vi "valves_flushrings.vi"(0 "COM4 in":refnum<k24>, 2 "Input solution":dbl=1.0, 3 "Rings to open":u32, 5 "error in":errorcluster) -> (6 "COM4 out":refnum<k24>, 8 "error out":errorcluster)   [LabVIEW 2018]
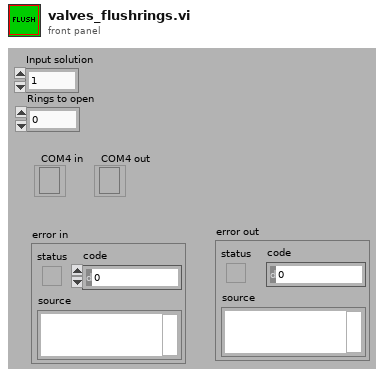
[diagram p1: front panel]
types:
  T1 = cluster{"Op A":u8[], "Op B":u8[], "Op C":u8[], "open":u8[], "L 3 A":u8[], "L 4 A 16":u8[], "F1 A":u8[], "L 4 A 34":u8[], "L 4 A 5":u8[], "FPw1 A":u8[], "L 2 A":u8[], "L 1 C FS":u8[], "L 2 C FS":u8[], "L 4 C 456 FS":u8[], "L 4 C 123 FS":u8[], "L 1 A":u8[], "L 1 C":u8[], "L 2 C":u8[], "L 4 C 456":u8[], "L 4 C 123":u8[], "FPw1 C":u8[], "F1 B":u8[], "F1 C":u8[], "F2 C":u8[], "F5 C":u8[]}
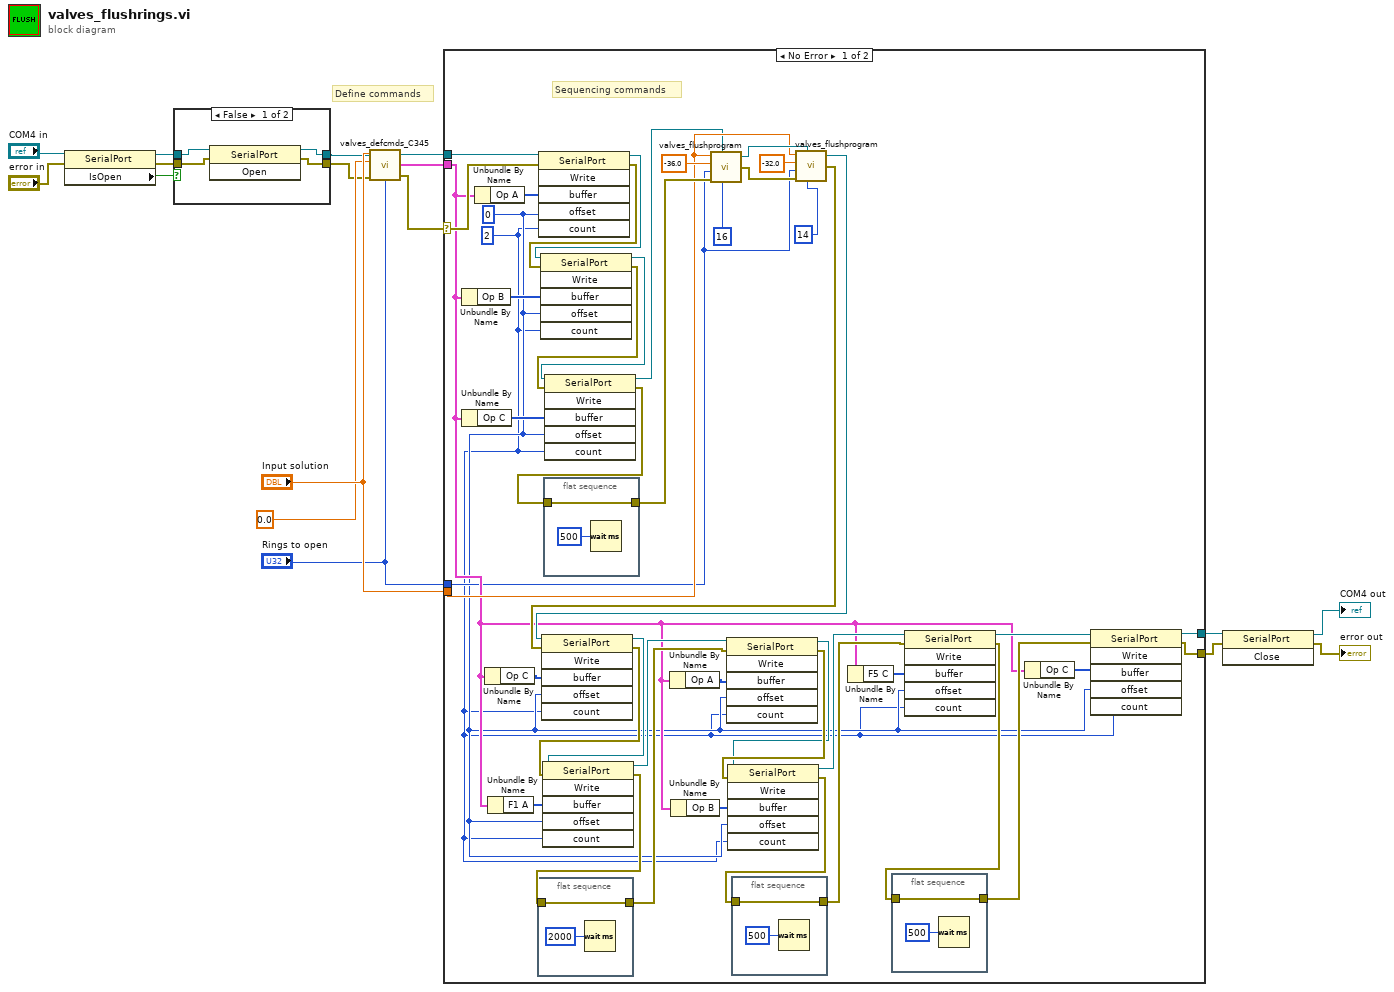
[diagram p0: block diagram]
diagram:
  # "Define commands"
  n1 = property class="SerialPort"(reference="COM4 in", error in="error in") -> (reference out=w9:refnum<k24>, error out=w10:errorcluster, "IsOpen"=w11:bool)
  n2 = case shown="False" w11 {
    tunnel: [w18 w23] -> w7
    tunnel: [w19 w22] -> w6
    tunnel: w10 -> [w20 w22]
    tunnel: w9 -> [w21 w23]
    frame False {
      n3 = invoke class="SerialPort" method="Open"(reference=w21, error in=w20) -> (reference out=w18:refnum<k24>, error out=w19:errorcluster)  [unwired: 1 in, 1 out]
    }
    frame True {
    }
  }
  n4 = call "valves_defcmds_C345.vi"("Input solution"="Input solution", "Add to C"=0.0, "Rings to open"="Rings to open", "error in"=w6, "COM4 in"=w7) -> ("COM4 out"=w15:refnum<k24>, "Commands out"=w16:T1, "error out"=w17:errorcluster)
  n5 = case shown="No Error" w17 {
    selector: w17 -> [w63 w79]
    tunnel: w15 -> [w69 w78]
    tunnel: [w54 w79] -> w4
    tunnel: w16 -> [w38 _]
    tunnel: "Rings to open" -> [w36 _]
    tunnel: "Input solution" -> [w43 _]
    tunnel: [w47 w78] -> w2
    frame No Error {
      w24 = 2 ("count")
      w25 = 0 ("offset")
      # "Sequencing commands"
      n6 = Unbundle By Name(w38) -> ("Op B"=w34:u8[])
      n7 = Unbundle By Name(w38) -> ("Op C"=w33:u8[])
      n8 = Unbundle By Name(w38) -> ("Op A"=w35:u8[])
      n9 = Unbundle By Name(w38) -> ("Op C"=w31:u8[])
      n10 = Unbundle By Name(w38) -> ("F1 A"=w26:u8[])
      n11 = flat-sequence {
        tunnel: [w74] -> w46
        tunnel: w45 -> [w74]
        frame #0 {
          n12 = Wait (ms)(milliseconds to wait=u32 2000) -> ()  [unwired: 1 out]
        }
      }
      n13 = invoke class="SerialPort" method="Write"(reference=w69, error in=w63, "buffer"=w35, "offset"=w25, "count"=w24) -> (reference out=w68:refnum<k24>, error out=w67:errorcluster)  [unwired: 1 in, 4 out]
      n14 = invoke class="SerialPort" method="Write"(reference=w68, error in=w67, "buffer"=w34, "offset"=w25, "count"=w24) -> (reference out=w66:refnum<k24>, error out=w65:errorcluster)  [unwired: 1 in, 4 out]
      n15 = flat-sequence {
        tunnel: [w76] -> w62
        tunnel: w64 -> [w76]
        frame #0 {
          n16 = Wait (ms)(milliseconds to wait=u32 500) -> ()  [unwired: 1 out]
        }
      }
      n17 = invoke class="SerialPort" method="Write"(reference=w66, error in=w65, "buffer"=w33, "offset"=w25, "count"=w24) -> (reference out=w32:refnum<k24>, error out=w64:errorcluster)  [unwired: 1 in, 4 out]
      n18 = Unbundle By Name(w38) -> ("Op A"=w30:u8[])
      n19 = Unbundle By Name(w38) -> ("Op B"=w27:u8[])
      n20 = call "valves_flushprogram.vi"("Input solution"=w43, "COM4 in"=w32, "Add to C"=-36.0, "Rings to open"=w36, "Cycles"=16 ("Input solution"), "error in"=w62) -> ("COM4 out"=w59:refnum<k24>, "error out"=w58:errorcluster)  [unwired: 1 in]
      n21 = flat-sequence {
        tunnel: [w72] -> w41
        tunnel: w42 -> [w72]
        frame #0 {
          n22 = Wait (ms)(milliseconds to wait=u32 500) -> ()  [unwired: 1 out]
        }
      }
      n23 = call "valves_flushprogram.vi"("Input solution"=w43, "COM4 in"=w59, "Add to C"=-32.0, "Rings to open"=w36, "Cycles"=14 ("Input solution"), "error in"=w58) -> ("COM4 out"=w53:refnum<k24>, "error out"=w57:errorcluster)  [unwired: 1 in]
      n24 = invoke class="SerialPort" method="Write"(reference=w53, error in=w57, "buffer"=w31, "offset"=w25, "count"=w24) -> (reference out=w52:refnum<k24>, error out=w56:errorcluster)  [unwired: 1 in, 4 out]
      n25 = invoke class="SerialPort" method="Write"(reference=w52, error in=w56, "buffer"=w26, "offset"=w25, "count"=w24) -> (reference out=w51:refnum<k24>, error out=w45:errorcluster)  [unwired: 1 in, 4 out]
      n26 = invoke class="SerialPort" method="Write"(reference=w51, error in=w46, "buffer"=w30, "offset"=w25, "count"=w24) -> (reference out=w50:refnum<k24>, error out=w55:errorcluster)  [unwired: 1 in, 4 out]
      n27 = invoke class="SerialPort" method="Write"(reference=w50, error in=w55, "buffer"=w27, "offset"=w25, "count"=w24) -> (reference out=w49:refnum<k24>, error out=w42:errorcluster)  [unwired: 1 in, 4 out]
      n28 = Unbundle By Name(w38) -> ("F5 C"=w29:u8[])
      n29 = flat-sequence {
        tunnel: [w70] -> w39
        tunnel: w40 -> [w70]
        frame #0 {
          n30 = Wait (ms)(milliseconds to wait=u32 500) -> ()  [unwired: 1 out]
        }
      }
      n31 = invoke class="SerialPort" method="Write"(reference=w49, error in=w41, "buffer"=w29, "offset"=w25, "count"=w24) -> (reference out=w48:refnum<k24>, error out=w40:errorcluster)  [unwired: 1 in, 4 out]
      n32 = Unbundle By Name(w38) -> ("Op C"=w28:u8[])
      n33 = invoke class="SerialPort" method="Write"(reference=w48, error in=w39, "buffer"=w28, "offset"=w25, "count"=w24) -> (reference out=w47:refnum<k24>, error out=w54:errorcluster)  [unwired: 1 in, 4 out]
    }
    frame Error {
    }
  }
  n34 = invoke class="SerialPort" method="Close"(reference=w2, error in=w4) -> (reference out=→"COM4 out":refnum<k24>, error out=→"error out":errorcluster)  [unwired: 1 in, 1 out]
